vi "API_DB.GetAllFullLocations.vi"(0 "Database in":refnum<class "Database.lvclass">, 1 "Wait (F)":bool, 5 "Table":string, 11 "error in (no error)":errorcluster, 12 "Timeout (ms)":u32) -> (4 "Database out":refnum<class "Database.lvclass">, 6 "Slot":string, 15 "error out":errorcluster)   [LabVIEW 2022 SP3]
doc: "Developed by Kevin Thompson\nkevin@thompsonengineering.net\n\nCopyright 2018\nThompson Engineering, LLC"
uses:
  Database.lvclass
  DataTypes/AsynCmd_Temp01--enum.ctl
  Database.lvclass/Database.ctl
  DataTypes/QuiryBuilderData--Cluster.ctl
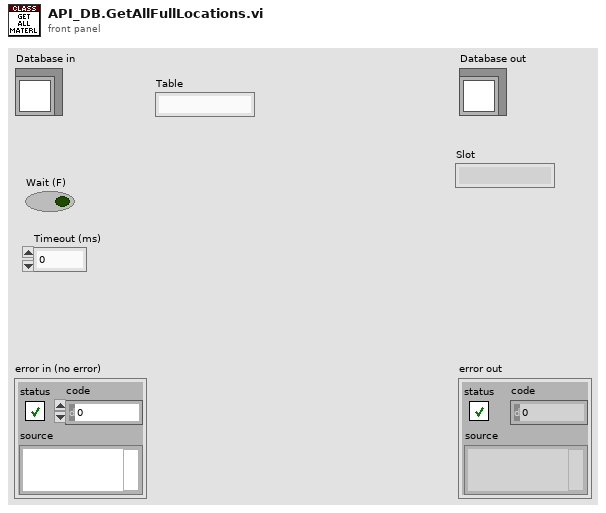
[diagram p1: front panel]
types:
  T1 = typedef "QuiryBuilderData--Cluster.ctl" = cluster{"Table":string, "Column":string[], "Value":string[], "WhereColumn":string[], "WhereValue":string[], "OrderBy":string[]}
  T2 = typedef "Database.lvclass/AsynCmd_Temp01--enum.ctl" = enum16{"DB.DeleteRecord", "DB.UpdateRecord", "DB.InsertRecord", "DB.SelectRecord", "DB.ExecuteSQLCommand", "DB.FindFirstSlot", "DB.GenericSQLQuery"}
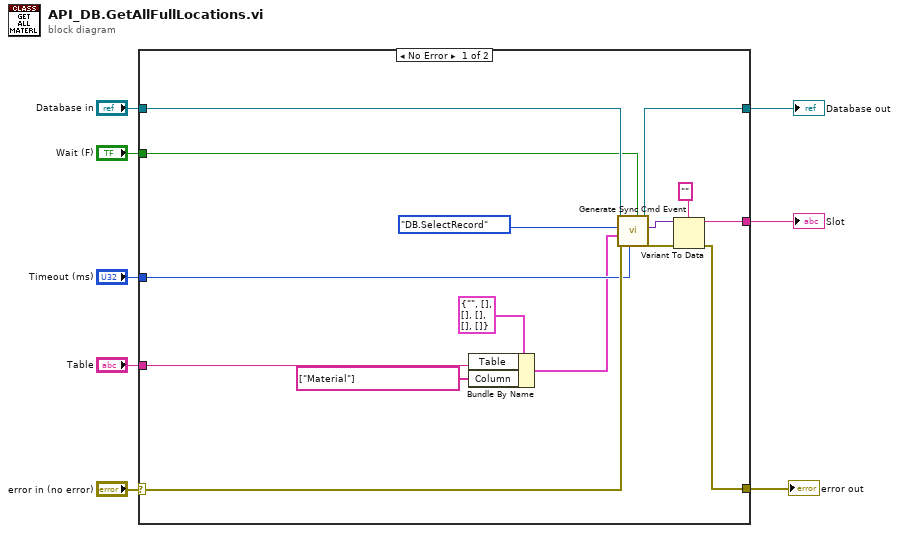
[diagram p0: block diagram]
diagram:
  n1 = case shown="No Error" "error in (no error)" {
    selector: "error in (no error)" -> [w21 w25]
    tunnel: [w16 w25] -> w7
    tunnel: [w22 w24] -> w5
    tunnel: "Database in" -> [w23 w24]
    tunnel: [w18 _] -> w2
    tunnel: "Wait (F)" -> [w15 _]
    tunnel: "Timeout (ms)" -> [w14 _]
    tunnel: "Table" -> [w11 _]
    frame No Error {
      n2 = Bundle By Name(cluster=T1 {"Table"="", "Column"=[], "Value"=[], "WhereColumn"=[], "WhereValue"=[], "OrderBy"=[]} ("QueryBuilderData"), "Table"=w11, "Column"=string[] ["Material"]) -> (w12:T1)
      n3 = call "Generate Sync Cmd Event.vi"("Wait (F)"=w15, "Timeout (ms)"=w14, "error in (no error)"=w21, "vData"=w12, "AsyncCmd"=AsynCmd_Temp01--enum."DB.SelectRecord", "Database in"=w23) -> ("error out"=w17:errorcluster, "Return Value"=w19:variant, "Database out"=w22:refnum<class "Database.lvclass">)  [unwired: 3 in]
      n4 = Variant To Data(error in=w17, type="", Variant=w19) -> (data=w18:string, error out=w16:errorcluster)
    }
    frame Error {
    }
  }
  "error out" <- w7
  "Database out" <- w5
  "Slot" <- w2
